vi "UDP - Data PID (SubVI).vi"(8 "error in (no error)":errorcluster, 11 "Data":string="\u0002X::\u0000ï²k7ªª5@%\u0019è?\u0000\u0000\u0000\u0000«\u0000\u0000\u0000ÈA\u0000\u0000\u0000\u0000\u000f\u0000\u0000\u0000ùÿÿÿDisp\u0000\u0000\u0000\u0000\u0000\u0000\u0000\u0000\u0000\u0000\u0000\u0000\u0000\u0000\u0000\u0000\u0000\u0000\u0000\u0000\u0000\u0000\u0000\u0000\u0000\u0000\u0000\u0000\u0000\u0000\u0000\u0000\u0000\u0000\u0000\u0000\u0000\u0000\u0000\u0000\u0000\u0000\u0000\u0000Â") -> (0 "error out":errorcluster, 3 "PID Setting":T1, 4 "Success":bool)   [LabVIEW 2019]
panel:
  in  "Data 2":string="\u0000\u0000;:\u0000ï²k7ªª5@%\u0019è?\u0000\u0000\u0000\u0000«\u0000\u0000\u0000ÈA\u0000\u0000\u0000\u0000\u000f\u0000\u0000\u0000\u0007\u0000\u0000\u0000Disp\u0000\u0000\u0000\u0000\u0000"
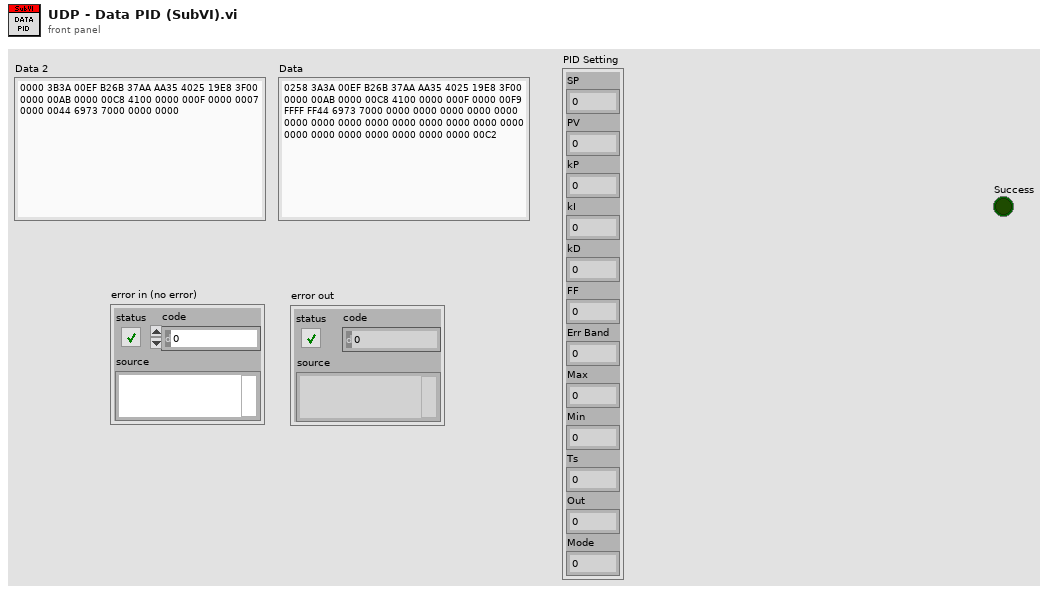
[diagram p1: front panel]
types:
  T1 = cluster{"SP":sgl, "PV":sgl, "kP":sgl, "kI":sgl, "kD":sgl, "FF":sgl, "Err Band":sgl, "Max":i32, "Min":i32, "Ts":u32, "Out":i32, "Mode":u8}
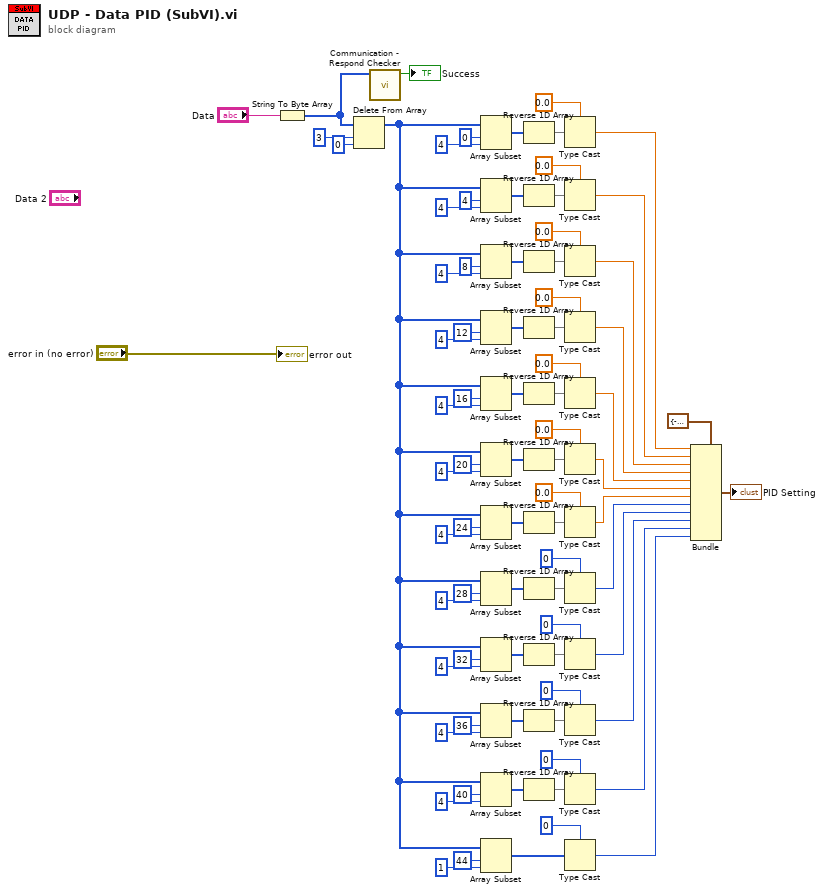
[diagram p0: block diagram]
diagram:
  n1 = String To Byte Array(string="Data") -> (unsigned byte array=w1:u8[])
  n2 = Delete From Array(array=w1, length=3, index=0) -> (array with subset deleted=w21:u8[])  [unwired: 1 out]
  n3 = call "Communication - Respond Checker.vi"("Read Data"=w1) -> ("Success"=→"Success":bool)  [unwired: 10 in]
  n4 = Array Subset(array=w21, index=0, length=4) -> (w75:u8[])
  n5 = Array Subset(array=w21, index=4, length=4) -> (w70:u8[])
  n6 = Array Subset(array=w21, index=8, length=4) -> (w65:u8[])
  n7 = Array Subset(array=w21, index=12, length=4) -> (w60:u8[])
  n8 = Array Subset(array=w21, index=16, length=4) -> (w55:u8[])
  n9 = Array Subset(array=w21, index=20, length=4) -> (w32:u8[])
  n10 = Array Subset(array=w21, index=24, length=4) -> (w37:u8[])
  n11 = Array Subset(array=w21, index=28, length=4) -> (w42:u8[])
  n12 = Array Subset(array=w21, index=32, length=4) -> (w47:u8[])
  n13 = Array Subset(array=w21, index=36, length=4) -> (w20:u8[])
  n14 = Array Subset(array=w21, index=40, length=4) -> (w27:u8[])
  n15 = Array Subset(array=w21, index=44, length=1) -> (w18:u8[])
  n16 = Reverse 1D Array(array=w75) -> (reversed array=w74:u8[])
  n17 = Reverse 1D Array(array=w70) -> (reversed array=w71:u8[])
  n18 = Reverse 1D Array(array=w65) -> (reversed array=w64:u8[])
  n19 = Reverse 1D Array(array=w60) -> (reversed array=w61:u8[])
  n20 = Reverse 1D Array(array=w55) -> (reversed array=w54:u8[])
  n21 = Reverse 1D Array(array=w32) -> (reversed array=w33:u8[])
  n22 = Reverse 1D Array(array=w37) -> (reversed array=w36:u8[])
  n23 = Reverse 1D Array(array=w42) -> (reversed array=w43:u8[])
  n24 = Reverse 1D Array(array=w47) -> (reversed array=w46:u8[])
  n25 = Reverse 1D Array(array=w20) -> (reversed array=w19:u8[])
  n26 = Reverse 1D Array(array=w27) -> (reversed array=w28:u8[])
  n27 = Type Cast(type=sgl 0.0, x=w74) -> (*(type *) &x=w16:sgl)
  n28 = Type Cast(type=sgl 0.0, x=w71) -> (*(type *) &x=w15:sgl)
  n29 = Type Cast(type=sgl 0.0, x=w64) -> (*(type *) &x=w14:sgl)
  n30 = Type Cast(type=sgl 0.0, x=w61) -> (*(type *) &x=w13:sgl)
  n31 = Type Cast(type=sgl 0.0, x=w54) -> (*(type *) &x=w12:sgl)
  n32 = Type Cast(type=sgl 0.0, x=w33) -> (*(type *) &x=w11:sgl)
  n33 = Type Cast(type=sgl 0.0, x=w36) -> (*(type *) &x=w10:sgl)
  n34 = Type Cast(type=0, x=w43) -> (*(type *) &x=w9:i32)
  n35 = Type Cast(type=0, x=w46) -> (*(type *) &x=w8:i32)
  n36 = Type Cast(type=u32 0, x=w19) -> (*(type *) &x=w7:u32)
  n37 = Type Cast(type=0, x=w28) -> (*(type *) &x=w6:i32)
  n38 = Type Cast(type=u8 0, x=w18) -> (*(type *) &x=w5:u8)
  n39 = Bundle(cluster=T1 {"SP"=-2.7823365e-08, "PV"=-3.023652e-13, "kP"=8.5432666e-24, "kI"=2.29252e-41, "kD"=1.570387e-38, "FF"=25.0, "Err Band"=0.0, "Max"=15, "Min"=-7, "Ts"=1886611780, "Out"=0, "Mode"=0}, "SP"=w16, "PV"=w15, "kP"=w14, "kI"=w13, "kD"=w12, "FF"=w11, "Err Band"=w10, "Max"=w9, "Min"=w8, "Ts"=w7, "Out"=w6, "Mode"=w5) -> (→"PID Setting":T1)
  "error out" <- "error in (no error)"
